vi "Read Autoshutdown_ (T).vi"(8 "error in (no error)":errorcluster, 11 "JQMHStartup in":refnum<class "JQMHStartup.lvclass">) -> (0 "error out":errorcluster, 2 "Autoshutdown? (T)":bool=TRUE, 3 "JQMHStartup out":refnum<class "JQMHStartup.lvclass">)   [LabVIEW 2024, in "JQMHStartup.lvclass"]
uses:
  JQMHStartup.lvclass
  JQMHStartup.lvclass/JQMHStartup.ctl
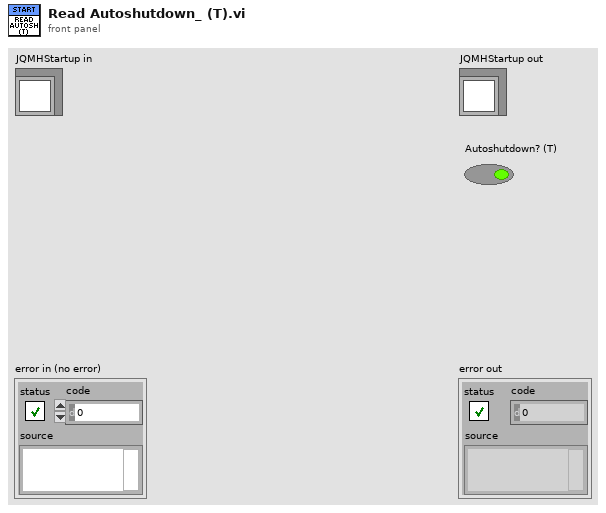
[diagram p1: front panel]
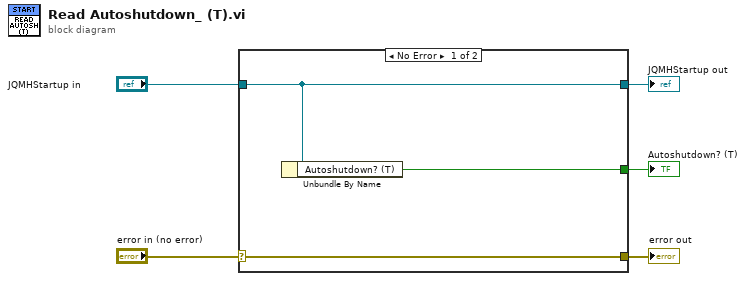
[diagram p0: block diagram]
diagram:
  n1 = case shown="No Error" "error in (no error)" {
    selector: "error in (no error)" -> [w8 w9]
    tunnel: [w8 w9] -> w4
    tunnel: [w7 w10] -> w2
    tunnel: "JQMHStartup in" -> [w7 w10]
    tunnel: [w6 _] -> w1
    frame No Error {
      n2 = Unbundle By Name(w7) -> ("Autoshutdown? (T)"=w6:bool)
    }
    frame Error {
    }
  }
  "error out" <- w4
  "JQMHStartup out" <- w2
  "Autoshutdown? (T)" <- w1
